vi "Read NI 9422 - Digital Input.vi"(8 "error in":errorcluster, 11 "NI 9422 in":refnum<class "NI 9422.lvclass">) -> (0 "error out":errorcluster, 2 "channel settings":T1[](array[typedef]), 3 "NI 9422 out":refnum<class "NI 9422.lvclass">)   [LabVIEW 2020, in "Scan Engine Scripting.lvlib" / "NI 9422.lvclass"]
doc: "Returns the channel settings of a NI-9422 digital input module that can be edited and then used to create a new module instance to set into a slot."
uses:
  NI 9422.lvclass
  Mode Classes/Controls/digital channel settings.ctl
  Scan Engine Scripting.lvlib
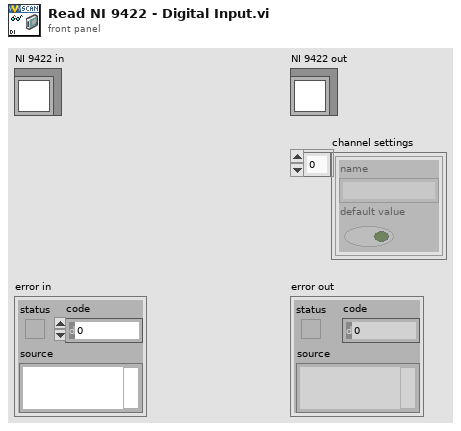
[diagram p1: front panel]
types:
  T1 = typedef "Scan Engine Scripting.lvlib/digital channel settings.ctl" = cluster{"name":string, "default value":bool}
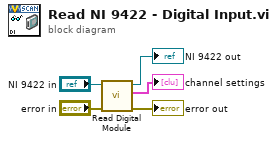
[diagram p0: block diagram]
diagram:
  n1 = call-dynamic "Read Digital Module.vi"("error in"="error in", "module in"="NI 9422 in") -> ("error out"=→"error out":errorcluster, "channel settings"=→"channel settings":T1[], "module out"=→"NI 9422 out":refnum<class "NI 9422.lvclass">)  [unwired: 7 in]
